vi "MAIN RS485.vi"(4 "message":string="help", 6 "CIB address":string="0", 8 "Error In":errorcluster, 9 "Timeout (ms)":u32=2000, 10 "RS485 Operation":u16(ring) items=["Initialize Port", "Send Command", "Get Commands"], 11 "PortConfig":T1={"VISA resource name"="COM7", "baud rate"=19200, "data bits (8)"=8, "parity (0:none)"=enum."None", "stop bits (10: 1 bit)"=10, "flow control (0:none)"=0, "timeout (2sec)"=2000} {"flow control (0:none)" items=["None", "XON/XOFF", "RTS/CTS", "XON/XOFF & RTS/CTS", "DTR/DSR", "XON/XOFF & DTR/DSR"]; "stop bits (10: 1 bit)" items=["1.0"=10, "1.5"=15, "2.0"=20]}) -> (0 "Error Out":errorcluster, 2 "Return String[]":string[](array[string]))   [LabVIEW 2013]
uses:
  Port Config.ctl
  <vilib>/Instr/_visa.llb/VISA Set IO Buffer Mask.ctl
  <vilib>/Instr/_visa.llb/VISA Configure Serial Port (Instr).vi
  <vilib>/Utility/error.llb/DialogType.ctl
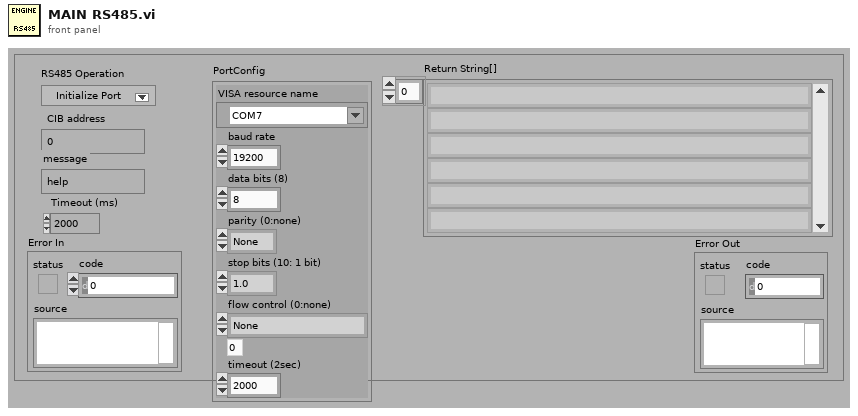
[diagram p1: front panel]
types:
  T1 = typedef "Port Config.ctl" = cluster{"VISA resource name":refnum<visa-resource-name>, "baud rate":u32, "data bits (8)":u16, "parity (0:none)":enum16{"None", "Odd", "Even", "Mark", "Space"}, "stop bits (10: 1 bit)":u16, "flow control (0:none)":u16, "timeout (2sec)":u32}
  T2 = cluster{"PortConfig":T1, "CIB address":string, "message":string, "Timeout (ms)":u32, "Error":errorcluster, "Return String[]":string[]}
  T3 = typedef "VISA Set IO Buffer Mask.ctl" = u16
  T4 = typedef "DialogType.ctl" = u16
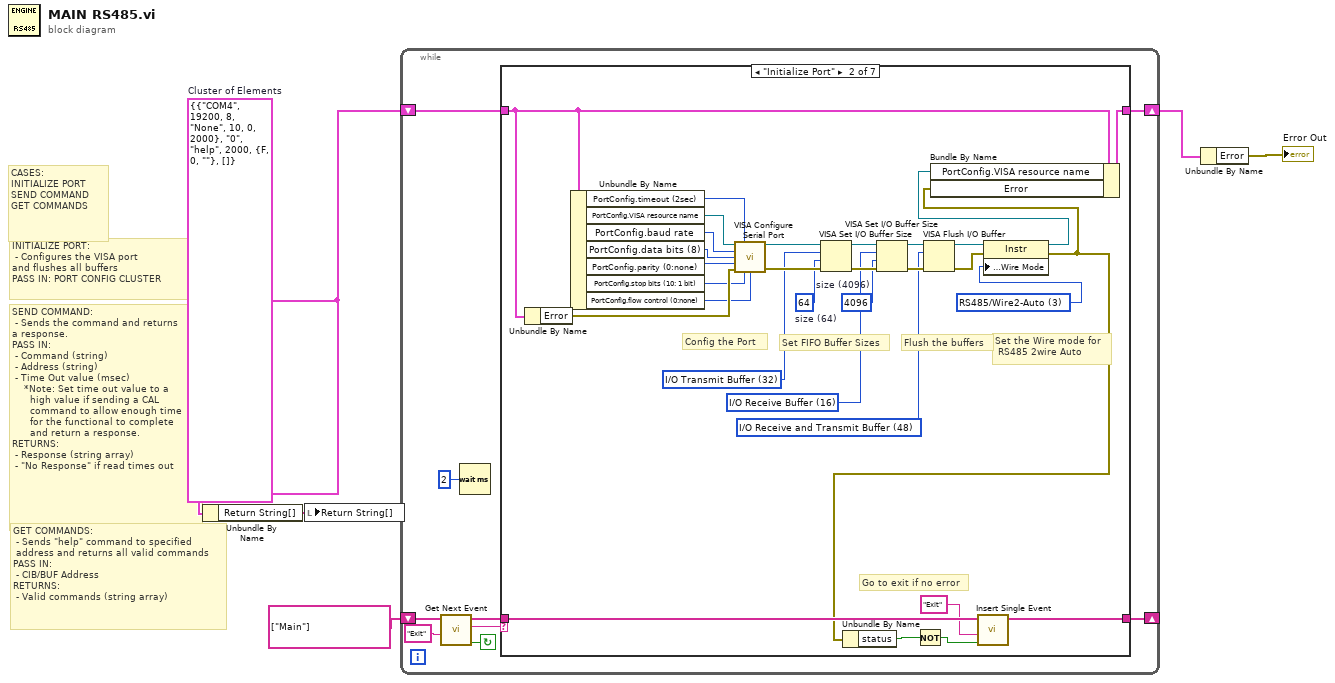
[diagram p0: block diagram]
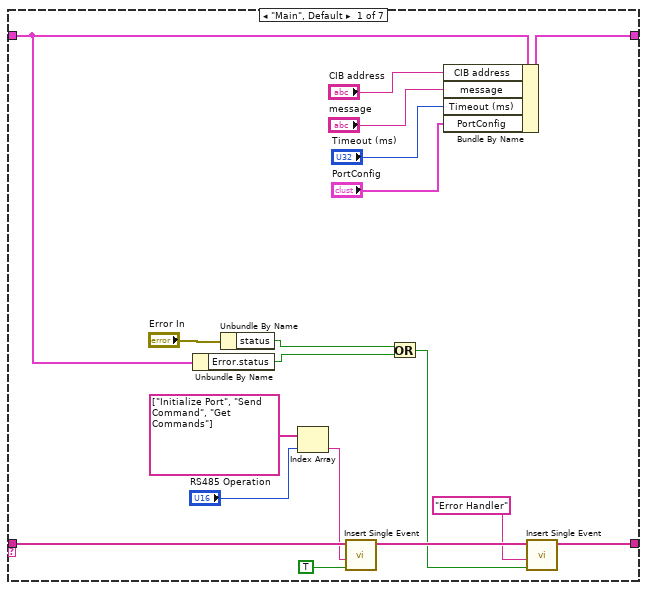
[diagram p2: hidden frame]
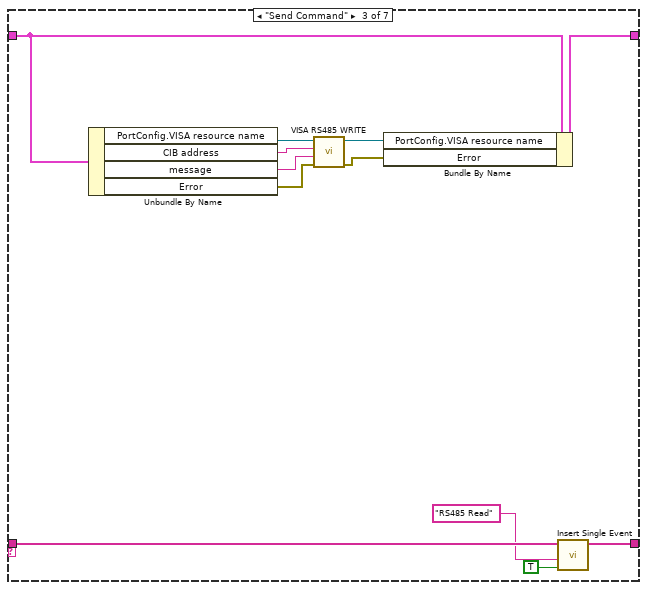
[diagram p3: hidden frame]
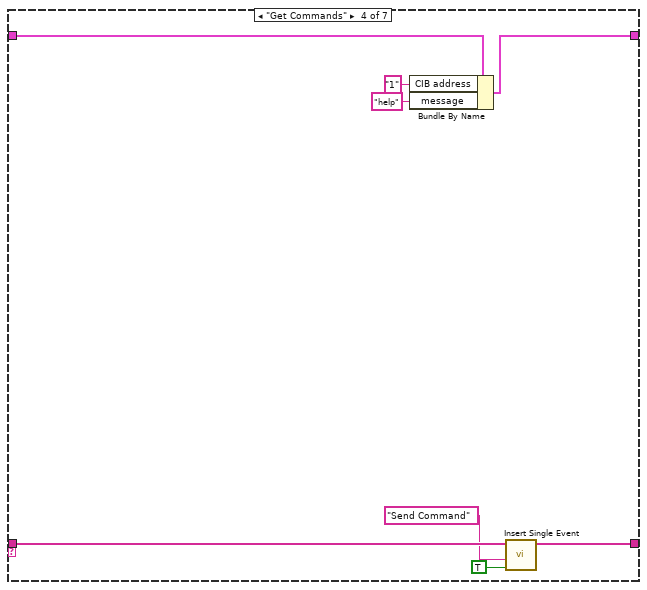
[diagram p4: hidden frame]
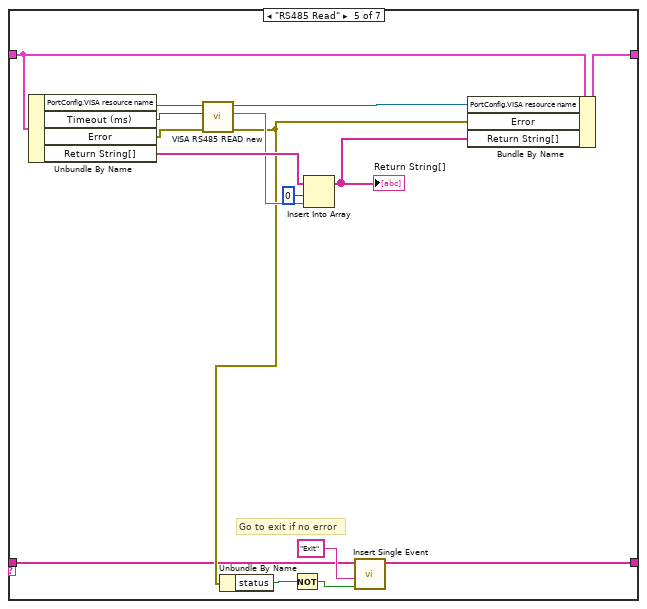
[diagram p5: hidden frame]
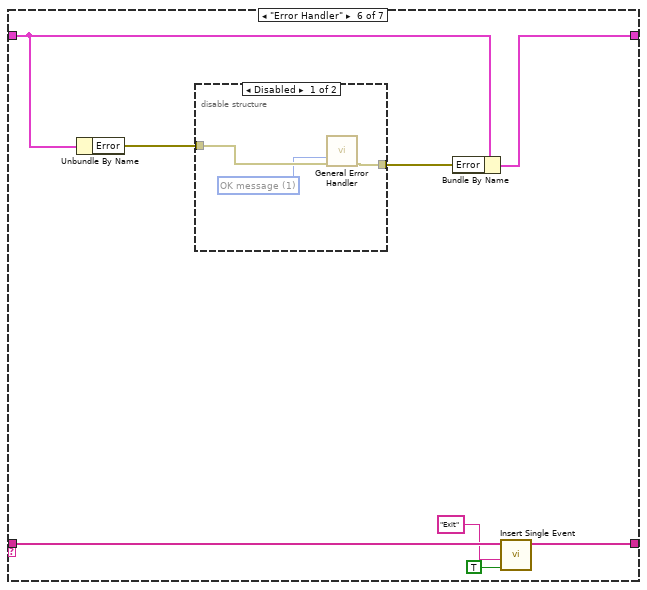
[diagram p6: hidden frame]
diagram:
  w2 = T2 {"PortConfig"={"VISA resource name"="COM4", "baud rate"=19200, "data bits (8)"=8, "parity (0:none)"=enum."None", "stop bits (10: 1 bit)"=10, "flow control (0:none)"=0, "timeout (2sec)"=2000}, "CIB address"="0", "message"="help", "Timeout (ms)"=2000, "Error"={"status"=FALSE, "code"=0, "source"=""}, "Return String[]"=[]}  # Cluster of Elements
  # "GET COMMANDS:\n - Sends \"help\" command to specified\n address and returns all valid commands\nPASS IN:\n - CIB/BUF Address\nRETURNS:\n - Valid commands (string array)"
  # "SEND COMMAND:\n - Sends the command and returns\na response.\nPASS IN:\n - Command (string)\n - Address (string)\n - Time Out value (msec)\n    *Note: Set time out value to a \n      high value if sending a CAL \n      command to allow enough time\n      for the functional to complete\n      and return a response.\nRETURNS:\n - Response (string array)\n - \"No Response\" if read times out"
  # "INITIALIZE PORT:\n - Configures the VISA port\nand flushes all buffers\nPASS IN: PORT CONFIG CLUSTER"
  # "CASES:\nINITIALIZE PORT\nSEND COMMAND\nGET COMMANDS"
  n1 = Unbundle By Name(w2) -> ("Return String[]"=w1:string[])
  n2 = local write "Return String[]"(w1) -> ()
  n3 = while {
    shift-left: string[] ["Main"] ("event queue out") -> [w12]
    shift-right: [w9] -> _
    shift-left: w2 -> [w6]
    shift-right: [w11] -> w4
    stop <- w14 continue-if-true
    n4 = call "Get Next Event.vi"("Exit Event"="Exit", "event queue in"=w12) -> ("Condition (Exit:F)"=w14:bool, "next event"=w13:string, "event queue out"=w10:string[])  [unwired: 3 out]
    n5 = Wait (ms)(milliseconds to wait=u32 2) -> ()  [unwired: 1 out]
    n6 = case shown="\"Initialize Port\"" w13 {
      tunnel: w6 -> [w24 w33 w70 w79 w99 w106 w113]
      tunnel: [w30 w63 w69 w78 w98 w105 w113] -> w11
      tunnel: [w22 w38 w66 w82 w84 w104 w112] -> w9
      tunnel: w10 -> [w32 w39 w75 w83 w85 w107 w112]
      frame "Main", Default {
        n7 = Unbundle By Name(w24) -> ("Error.status"=w19:bool)
        n8 = Unbundle By Name("Error In") -> ("status"=w20:bool)
        n9 = Index Array(array=string[] ["Initialize Port", "Send Command", "Get Commands"] ("Events to Insert"), index="RS485 Operation") -> (element=w25:string)
        n10 = call "Insert Single Event.vi"("Insert?"=TRUE ("Insert all? (T)"), "Event to insert"=w25, "Event queue in"=w32) -> ("Event queue out"=w23:string[])  [unwired: 1 in, 3 out]
        n11 = Or(x=w20, y=w19) -> (x .or. y?=w18:bool)
        n12 = Bundle By Name(cluster=w24, "CIB address"="CIB address", "message"="message", "Timeout (ms)"="Timeout (ms)", "PortConfig"="PortConfig") -> (w30:T2)
        n13 = call "Insert Single Event.vi"("Insert?"=w18, "Event to insert"="Error Handler", "Event queue in"=w23) -> ("Event queue out"=w22:string[])  [unwired: 4 out]
      }
      frame "Initialize Port" {
        w42 = u32 4096  # size (4096)
        w43 = u32 64  # size (64)
        w44 = T3 32 items=["I/O Receive Buffer"=16, "I/O Transmit Buffer"=32, "I/O Receive and Transmit Buffer"=48] ("Mask")
        w41 = T3 16 items=["I/O Receive Buffer"=16, "I/O Transmit Buffer"=32, "I/O Receive and Transmit Buffer"=48] ("Mask")
        w40 = T3 48 items=["I/O Receive Buffer"=16, "I/O Transmit Buffer"=32, "I/O Receive and Transmit Buffer"=48] ("Mask")
        w57 = i16 3 items=["Unknown"=-1, "RS485/Wire4"=0, "RS485/Wire2-EchoDTR"=1, "RS485/Wire2-CtrlDTR"=2, "RS485/Wire2-Auto"=3, "RS232/DTE"=128, "RS232/DCE"=129, "RS232/AUTO"=130] ("Serial Settings:Wire Mode")
        # "Go to exit if no error"
        # "Config the Port"
        # "Set the Wire mode for\n RS485 2wire Auto"
        # "Flush the buffers"
        # "Set FIFO Buffer Sizes"
        n14 = Unbundle By Name(w33) -> ("Error"=w56:errorcluster)
        n15 = Unbundle By Name(w33) -> ("PortConfig.timeout (2sec)"=w55:u32, "PortConfig.VISA resource name"=w54:refnum<visa-resource-name>, "PortConfig.baud rate"=w53:u32, "PortConfig.data bits (8)"=w52:u16, "PortConfig.parity (0:none)"=w51:enum16{"None", "Odd", "Even", "Mark", "Space"}, "PortConfig.stop bits (10: 1 bit)"=w50:u16, "PortConfig.flow control (0:none)"=w49:u16)
        n16 = call-poly "VISA Configure Serial Port"("VISA resource name"=w54, "timeout (10sec)"=w55, "baud rate (9600)"=w53, "data bits (8)"=w52, "parity (0:none)"=w51, "error in (no error)"=w56, "stop bits (10: 1 bit)"=w50, "flow control (0:none)"=w49) -> ("VISA resource name out"=w48:refnum<visa-resource-name>, "error out"=w47:errorcluster)  [unwired: 6 out]
        n17 = VISA Set I/O Buffer Size(VISA resource name=w48, mask (16)=w44, size (4096)=w43, error in (no error)=w47) -> (VISA resource name out=w45:refnum<visa-resource-name>, error out=w46:errorcluster)
        n18 = VISA Set I/O Buffer Size(VISA resource name=w45, mask (16)=w41, size (4096)=w42, error in (no error)=w46) -> (VISA resource name out=w60:refnum<visa-resource-name>, error out=w61:errorcluster)
        n19 = VISA Flush I/O Buffer(VISA resource name=w60, mask (16)=w40, error in (no error)=w61) -> (VISA resource name out=w59:refnum<visa-resource-name>, error out=w58:errorcluster)
        n20 = property class="Instr"(reference=w59, error in=w58, "Serial Settings:Wire Mode"=w57) -> (reference out=w62:refnum<visa-resource-name>, error out=w36:errorcluster)
        n21 = Unbundle By Name(w36) -> ("status"=w35:bool)
        n22 = Not(x=w35) -> (.not. x?=w34:bool)
        n23 = Bundle By Name(cluster=w33, "PortConfig.VISA resource name"=w62, "Error"=w36) -> (w63:T2)
        n24 = call "Insert Single Event.vi"("Insert?"=w34, "Event to insert"="Exit", "Event queue in"=w39) -> ("Event queue out"=w38:string[])  [unwired: 4 out]
      }
      frame "Send Command" {
        n25 = Unbundle By Name(w70) -> ("PortConfig.VISA resource name"=w74:refnum<visa-resource-name>, "CIB address"=w73:string, "message"=w72:string, "Error"=w71:errorcluster)
        n26 = call "VISA RS485 WRITE.vi"("error in (no error)"=w71, "message"=w72, "CIB address"=w73, "VISA resource name"=w74) -> ("error out"=w67:errorcluster, "dup VISA resource name"=w68:refnum<visa-resource-name>)  [unwired: 5 out]
        n27 = Bundle By Name(cluster=w70, "PortConfig.VISA resource name"=w68, "Error"=w67) -> (w69:T2)
        n28 = call "Insert Single Event.vi"("Insert?"=TRUE, "Event to insert"="RS485 Read", "Event queue in"=w75) -> ("Event queue out"=w66:string[])  [unwired: 4 out]
      }
      frame "Get Commands" {
        n29 = Bundle By Name(cluster=w79, "CIB address"="1", "message"="help") -> (w78:T2)
        n30 = call "Insert Single Event.vi"("Insert?"=TRUE, "Event to insert"="Send Command", "Event queue in"=w83) -> ("Event queue out"=w82:string[])  [unwired: 4 out]
      }
      frame "RS485 Read" {
        # "Go to exit if no error"
        n31 = Unbundle By Name(w99) -> ("PortConfig.VISA resource name"=w97:refnum<visa-resource-name>, "Timeout (ms)"=w94:u32, "Error"=w96:errorcluster, "Return String[]"=w93:string[])
        n32 = call "VISA RS485 READ new.vi"("error in (no error)"=w96, "Timeout (ms)"=w94, "VISA resource name"=w97) -> ("error out"=w86:errorcluster, "Return String"=w91:string, "dup VISA resource name"=w95:refnum<visa-resource-name>)  [unwired: 6 out]
        n33 = Unbundle By Name(w86) -> ("status"=w88:bool)
        n34 = Not(x=w88) -> (.not. x?=w87:bool)
        n35 = Insert Into Array(array=w93, index=0, new element=w91) -> (w90:string[])
        "Return String[]" <- w90
        n36 = call "Insert Single Event.vi"("Insert?"=w87, "Event to insert"="Exit", "Event queue in"=w85) -> ("Event queue out"=w84:string[])  [unwired: 4 out]
        n37 = Bundle By Name(cluster=w99, "PortConfig.VISA resource name"=w95, "Error"=w86, "Return String[]"=w90) -> (w98:T2)
      }
      frame "Error Handler" {
        n38 = Unbundle By Name(w106) -> ("Error"=w101:errorcluster)
        n39 = disable-structure shown="Disabled" {
          disable-tunnel: w101 -> [w110 w111]
          disable-tunnel: [w109 w111] -> w100
          frame Disabled {
            w108 = T4 1 items=["no dialog", "OK message", "continue or stop message", "OK message + warnings", "continue/stop + warnings"] ("type of dialog (OK msg:1)")
            n40 = call <vilib>:"General Error Handler.vi"("type of dialog (OK msg:1)"=w108, "error in (no error)"=w110) -> ("error out"=w109:errorcluster)  [unwired: 13 out]
          }
          frame Enabled {
          }
        }
        n41 = Bundle By Name(cluster=w106, "Error"=w100) -> (w105:T2)
        n42 = call "Insert Single Event.vi"("Insert?"=TRUE, "Event to insert"="Exit", "Event queue in"=w107) -> ("Event queue out"=w104:string[])  [unwired: 4 out]
      }
      frame "Exit" {
        # "This case will only run once before Exiting the program.\n\nThe Exit checker in the lower left of the While loop will stop the while loop after this loops execution."
      }
    }
  }
  n43 = Unbundle By Name(w4) -> ("Error"=→"Error Out":errorcluster)
